vi "SVFA Power Spectrum Subset (1 Ch).vi"(0 "scaled signal [EU]":waveform(dbl)={"t0"=timestamp(0 s since 1904-01-01), "dt"=1e-05, "Y"=[]}, 2 "window":T7=1 items=["None"=0, "Hanning"=1, "Hamming"=2, "Blackman-Harris"=3, "Exact Blackman"=4, "Blackman"=5, "Flat Top"=6, "4 Term B-Harris "=7, "7 Term B-Harris"=8, "Low Sidelobe"=9, "Force"=64, "Exponential"=65, "Blackman Nuttall"=11, "Triangle"=30, "Bartlett-Hanning"=31, "Bohman"=32, "Parzen"=33, "Welch"=34, "Kaiser"=60, "Dolph-Chebyshev"=61, "Gaussian"=62], 3 "frequency range":T9={"start frequency"=1000.0, "stop frequency"=2000.0} {"stop frequency" min=0.0 format="%.2f"; "start frequency" min=0.0 format="%.2f"}, 4 "dB On (T)":bool=TRUE, 5 "error in (no error)":errorcluster, 7 "averaging parameters":T8={"averaging mode"=enum."No averaging", "weighting mode"=enum."Exponential", "number of averages"=10, "linear mode"=enum."One shot"}, 9 "restart averaging (F)":bool) -> (11 "averaging done":bool, 13 "averages completed":dbl, 14 "power spectrum [dB EU]":cluster{"f0":dbl, "df":dbl, "magnitude":dbl[]}={"f0"=nan, "df"=inf, "magnitude"=[]} {"magnitude" format="%.2p"; "df" format="%.2p"; "f0" format="%.2p"}, 15 "unit label":string, 18 "spectrum info":T1={"channel name"="", "description"="", "x-axis units"=1, "spectral info"={"spectrum type"=enum."Power [Magnitude^2]", "linear/dB"=enum."linear", "window"=0, "window size"=0, "FFT size"=0}, "engineering units"=0, "custom label"="", "dB reference [EU]"=0.0, "peak units"=enum."rms", "weighting filter"=0, "spectral density?"=FALSE, "unit label"="", "spectrum skewed?"=FALSE, "complimentary spectrum units"=enum."none"} {"x-axis units" items=["Time (s)"=0, "Frequency-CB (Hz)"=1, "Frequency-CPB (Hz)"=1248, "Frequency-Arbitrary (Hz)"=2357, "Quefrency (s)"=2, "Revolutions (rev)"=3, "Order"=4, "Speed (RPM)"=11, "Speed (rad/s)"=21, "Index"=65535]; "weighting filter" items=["Linear", "A-weighting", "B-weighting", "C-weighting", "ITU-R 468-4", "Dolby", "CCITT", "C-message", "Wb", "Wc", "Wd", "We", "Wf", "Wh", "Wj", "Wk", "Wm", "AES17 20 kHz lowpass", "AES17 40 kHz lowpass", "AES17 20 kHz highpass", "AES17 40 kHz highpass"]; "dB reference [EU]" format="%.2f"; "engineering units" items=["custom..."=0, "V"=1, "A"=21, "C"=30, "pC"=31, "s"=32, "-"=29, "Pa"=2, "N"=20, "g"=3, "m/s^2"=4, "m/s"=5, "m"=6, "mm/s"=12, "mm"=13, "micron/s"=14, "micron"=15, "in/s^2"=7, "in/s"=8, "in"=9, "mil/s"=10, "mil"=11, "rad/s^2"=16, "rad/s"=17, "rad"=18, "deg/s^2"=26, "deg/s"=27, "deg"=28, "RPM"=22, "cycle/s^2"=23, "Hz"=24, "cycle"=25, "strain"=19]; "spectral info"."window" items=["None "=0, "Hanning"=1, "Hamming"=2, "Blackman-Harris"=3, "Exact Blackman"=4, "Blackman"=5, "Flat Top"=6, "4 Term B-Harris "=7, "7 Term B-Harris"=8, "Low Sidelobe"=9, "Force - Exponential"=10, "Gaussian"=62]}, 19 "error out":errorcluster)   [LabVIEW 2017]
doc: "Computes a subset of the power spectrum of <B>scaled signal [EU]</B>. The subset is defined by <B>frequency range</B>. Each block of data corresponds to a single FFT block and has to be passed individually to this VI. Wire data to the <B>scaled signal [EU]</B> input to determine the polymorphic instance to use or manually select the instance."
uses:
  <vilib>/addons/_NISVFA/_Shared subVIs/Controls/svc_Window.ctl
  <vilib>/addons/_NISVFA/_Shared subVIs/Controls/svc_Spectrum Info.ctl
  <vilib>/addons/_NISVFA/_Shared subVIs/Controls/svc_X-Axis Units.ctl
  <vilib>/addons/_NISVFA/_Shared subVIs/Controls/svc_Spectrum Type.ctl
  <vilib>/addons/_NISVFA/_Shared subVIs/Controls/svc_Engineering Units Text Ring.ctl
  <vilib>/addons/_NISVFA/_Shared subVIs/Controls/svc_Weighting Filter Text Ring.ctl
  <vilib>/addons/_NISVFA/_Shared subVIs/Controls/svc_Complimentary Spectrum Units.ctl
  <vilib>/addons/_NISVFA/_Shared subVIs/Spectrum Averaging/svfa_Reset Averaging State Info.vi
  <vilib>/addons/_NISVFA/_Shared subVIs/Spectrum Averaging/svfa_Average Array with Avg Checks (complex) No State.vi
  <vilib>/addons/_NISVFA/_Shared subVIs/Common/svc_Complex to Mag2 Array.vi
  <vilib>/addons/_NISVFA/_Shared subVIs/Spectrum Averaging/svfa_Average Array with Avg Checks (real) No State.vi
  <vilib>/addons/_NISVFA/_Shared subVIs/Windowing/svfa_Scaled Time Domain Window (Array).vi
  <vilib>/addons/_NISVFA/_Shared subVIs/Common/svc_Get SV Channel Info.vi
  <vilib>/addons/_NISVFA/_Shared subVIs/Common/svc_Spectrum Units.vi
  <vilib>/addons/_NISVFA/_Shared subVIs/Spectrum Averaging/svfa_Average Array (complex) No State.vi
  <vilib>/addons/_NISVFA/_Shared subVIs/Spectrum Averaging/svfa_Average Array (real) No State.vi
  <vilib>/Analysis/4window.llb/Force Window.vi
  <vilib>/Analysis/4window.llb/Force Window (DBL).vi
  <vilib>/Analysis/4window.llb/Exponential Window.vi
  <vilib>/Analysis/4window.llb/Exponential Window (DBL).vi
  <vilib>/addons/_NISVFA/_Shared subVIs/Spectrum Averaging/svfa_No Average Array (complex).vi
  <vilib>/addons/_NISVFA/_Shared subVIs/Spectrum Averaging/svfa_Average Array (complex).vi
  <vilib>/addons/_NISVFA/_Shared subVIs/Spectrum Averaging/svfa_No Average Array (real).vi
  <vilib>/addons/_NISVFA/_Shared subVIs/Spectrum Averaging/svfa_Average Array (real).vi
  <vilib>/addons/_NISVFA/_Shared subVIs/Spectrum Averaging/svfa_Peak Hold Array.vi
  <vilib>/addons/_NISVFA/_Shared subVIs/Common/svc_Get Weighting Enum and Labels.vi
  <vilib>/addons/_NISVFA/_Shared subVIs/Common/svc_Unit Label Lexical Class.vi
  <vilib>/addons/_NISVFA/_Shared subVIs/Common/svc_Engineering Units to Unit Label.vi
  <vilib>/addons/_NISVFA/_Shared subVIs/Common/svc_Format Value (DBL).vi
  <vilib>/addons/_NISVFA/_Shared subVIs/Common/svc_Channel Info to Spectrum Info.vi
  <vilib>/addons/_NISVFA/_Shared subVIs/Common/svc_Unit Label to Engineering Units.vi
  <vilib>/Utility/error.llb/Error Cluster From Error Code.vi
  <vilib>/Analysis/0measdsp.llb/Scaled Time Domain Window.vi
  <vilib>/Analysis/0measdsp.llb/Scaled Time Domain Window (DBL).vi
  <vilib>/addons/_NISVFA/_Spectrum Processing/subVIs/svfa_Spectrum Info Window to windowTd Type Def.vi
  <vilib>/addons/_NISVFA/_Shared subVIs/Common/svc_Window Parameters.vi
  <vilib>/addons/_NISVFA/_Shared subVIs/Common/svc_Get Window Info.vi
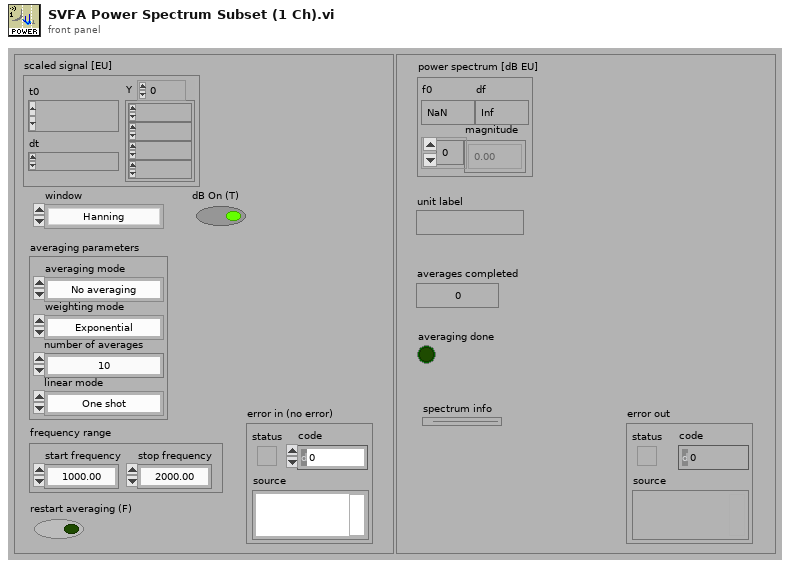
[diagram p1: front panel]
types:
  T1 = typedef "svc_Spectrum Info.ctl" = cluster{"channel name":string, "description":string, "x-axis units":T2, "spectral info":cluster{"spectrum type":T3, "linear/dB":enum16{"linear", "dB"}, "window":u16, "window size":i32, "FFT size":i32}, "engineering units":T4, "custom label":string, "dB reference [EU]":dbl, "peak units":enum16{"rms", "peak", "peak-peak"}, "weighting filter":T5, "spectral density?":bool, "unit label":string, "spectrum skewed?":bool, "complimentary spectrum units":T6}
  T2 = typedef "svc_X-Axis Units.ctl" = u16
  T3 = typedef "svc_Spectrum Type.ctl" = enum16{"FFT Spectrum [complex]", "Amplitude [Magnitude]", "Power [Magnitude^2]", "Cross Spectrum [complex]", "Frequency Response [Complex]"}
  T4 = typedef "svc_Engineering Units Text Ring.ctl" = u16
  T5 = typedef "svc_Weighting Filter Text Ring.ctl" = u16
  T6 = typedef "svc_Complimentary Spectrum Units.ctl" = enum16{"none", "radians", "degrees", "cycles", "imaginary"}
  T7 = typedef "svc_Window.ctl" = u32
  T8 = cluster{"averaging mode":enum16{"No averaging", "Vector averaging", "RMS averaging", "Peak hold"}, "weighting mode":enum16{"Linear", "Exponential"}, "number of averages":u32, "linear mode":enum16{"One shot", "Auto restart"}}
  T9 = cluster{"start frequency":dbl, "stop frequency":dbl}
  T10 = enum16{"Restart processing", "Continue processing", "Skip processing"}
  T11 = enum16{"No averaging", "Vector averaging", "RMS averaging", "Peak hold"}
  T12 = cluster{"complex FFT":cdb[], "real FFT":dbl[], "f0":dbl, "df":dbl, "averages completed":dbl, "averaging parameters":cluster{"averaging mode":enum16{"No averaging", "Vector averaging", "RMS averaging", "Peak hold"}, "weighting mode":enum16{"Linear", "Exponential"}, "number of averages":u32, "linear mode":enum16{"One shot", "Auto restart"}}}
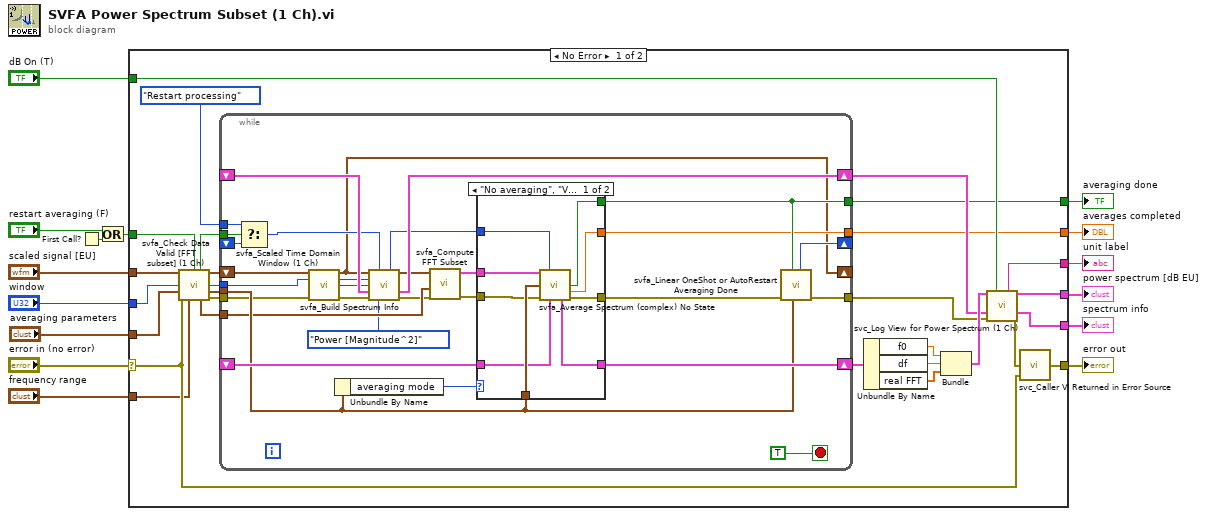
[diagram p0: block diagram]
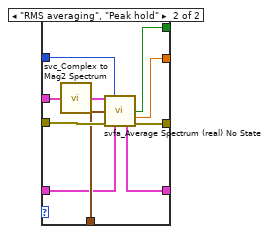
[diagram p2: hidden frame]
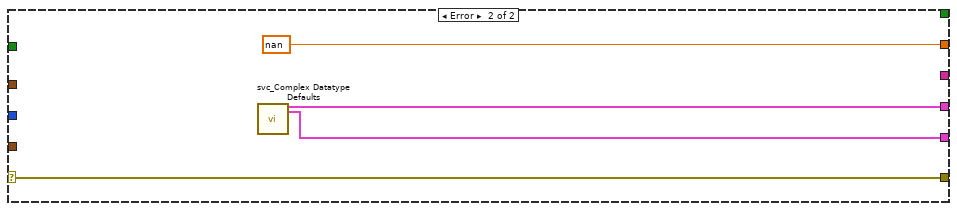
[diagram p3: hidden frame]
diagram:
  n1 = First Call?() -> (First Call?: T/F=w3:bool)
  n2 = Or(x="restart averaging (F)", y=w3) -> (x .or. y?=w2:bool)
  n3 = case shown="No Error" "error in (no error)" {
    selector: "error in (no error)" -> [w33 w96]
    tunnel: w2 -> [w41 _]
    tunnel: [w17 nan ("Averaged So-far")] -> w15
    tunnel: [w18 _] -> w14
    tunnel: [w38 w93] -> w9
    tunnel: [w35 w96] -> w13
    tunnel: "averaging parameters" -> [w40 _]
    tunnel: "frequency range" -> [w20 _]
    tunnel: "scaled signal [EU]" -> [w43 _]
    tunnel: "window" -> [w42 _]
    tunnel: [w37 _] -> w6
    tunnel: "dB On (T)" -> [w39 _]
    tunnel: [w34 w94] -> w4
    frame No Error {
      n4 = call <vilib>:"svfa_Check Data Valid [FFT subset] (1 Ch).vi"("signal"=w43, "restart averaging (F)"=w41, "window"=w42, "averaging parameters"=w40, "error in (no error)"=w33, "frequency range in"=w20) -> ("restart averaging"=w22:bool, "dup signal"=w28:waveform(dbl), "window"=w27:u16, "dup averaging parameters"=w24:T8, "frequency range out"=w19:T9, "error out"=w23:errorcluster)  [unwired: 4 in]
      n5 = while {
        shift-left: _ -> [w65]
        shift-right: [w66] -> w29
        tunnel: [w71] -> w17
        tunnel: [w72] -> w18
        tunnel: [w73] -> w16
        tunnel: w27 -> [w70]
        shift-right: [w68] -> w25
        shift-left: _ -> [w67]
        shift-right: [w64] -> _
        shift-left: _ -> [w63]
        tunnel: w24 -> [w61]
        tunnel: w23 -> [w60]
        tunnel: w22 -> [w59]
        tunnel: T10."Restart processing" ("t") -> [w58]
        tunnel: w19 -> [w57]
        shift-right: [w44] -> _
        shift-left: w28 -> [w45]
        stop <- TRUE stop-if-true
        n6 = Select(t=w58, s=w59, f=w63) -> (s? t:f=w62:T10)
        n7 = call <vilib>:"svfa_Scaled Time Domain Window (1 Ch).vi"("Signal in [X]"=w45, "window"=w70, "error in"=w60) -> ("Windowed Waveform"=w44:waveform(dbl), "dup window"=w49:T7, "window length"=w48:i32, "error out"=w50:errorcluster)  [unwired: 7 in, 2 out]
        n8 = Unbundle By Name(w61) -> ("averaging mode"=w56:T11)
        n9 = call <vilib>:"svfa_Build Spectrum Info.vi"("scaled signal [EU]"=w44, "processing control"=w62, "window"=w49, "window size"=w48, "spectrum info in"=w67, "error in (no error)"=w50, "spectrum type"=svc_Spectrum_Type."Power [Magnitude^2]" ("spectrum type 2")) -> ("dup processing control"=w47:T10, "dup scaled signal [EU]"=w46:waveform(dbl), "spectrum info out"=w68:T1, "error out"=w54:errorcluster)  [unwired: 5 in]
        n10 = call <vilib>:"svfa_Compute FFT Subset.vi"("error in (no error)"=w54, "frequency range"=w57, "windowed signal"=w46) -> ("error out"=w52:errorcluster, "FFT spectrum [Vrms]"=w51:cluster{"f0":dbl, "df":dbl, "spectrum":cdb[]})  [unwired: 7 in]
        n11 = case shown="\"No averaging\", \"Vector averaging\"" w56 {
          tunnel: w61 -> [w81 w86]
          tunnel: [w74 w83] -> w66
          tunnel: [w79 w90] -> w55
          tunnel: w51 -> [w82 w88]
          tunnel: w52 -> [w80 w92]
          tunnel: w47 -> [w76 w85]
          tunnel: [w77 w89] -> w71
          tunnel: w65 -> [w75 w84]
          tunnel: [w78 w91] -> w72
          frame "No averaging", "Vector averaging" {
            n12 = call <vilib>:"svfa_Average Spectrum (complex) No State.vi"("spectrum"=w82, "processing control"=w76, "averaging parameters"=w81, "error in (no error)"=w80, "averaging state info in"=w75) -> ("averaging done"=w78:bool, "averages completed"=w77:dbl, "averaging state info out"=w74:T12, "error out"=w79:errorcluster)  [unwired: 5 in, 2 out]
          }
          frame "RMS averaging", "Peak hold" {
            n13 = call <vilib>:"svc_Complex to Mag2 Spectrum.vi"("complex spectrum"=w88) -> ("power spectrum"=w87:cluster{"f0":dbl, "df":dbl, "spectrum":dbl[]})  [unwired: 4 in]
            n14 = call <vilib>:"svfa_Average Spectrum (real) No State.vi"("spectrum"=w87, "processing control"=w85, "averaging parameters"=w86, "error in (no error)"=w92, "averaging state info in"=w84) -> ("averaging done"=w91:bool, "averages completed"=w89:dbl, "averaging state info out"=w83:T12, "error out"=w90:errorcluster)  [unwired: 5 in, 2 out]
          }
        }
        n15 = call <vilib>:"svfa_Linear OneShot or AutoRestart Averaging Done.vi"("averaging parameters"=w61, "averaging done"=w72, "error in (no error)"=w55) -> ("error out"=w73:errorcluster, "processing control"=w64:T10)  [unwired: 7 in]
      }
      n16 = Unbundle By Name(w29) -> ("f0"=w32:dbl, "df"=w31:dbl, "real FFT"=w30:dbl[])
      n17 = Bundle("f0"=w32, "df"=w31, "real FFT"=w30) -> (w26:cluster{"f0":dbl, "df":dbl, "real FFT":dbl[]})  [unwired: 1 in]
      n18 = call <vilib>:"svc_Log View for Power Spectrum (1 Ch).vi"("power spectrum [dB EU]"=w26, "dB On (T)"=w39, "spectrum info"=w25, "error in (no error)"=w16) -> ("unit label"=w37:string, "power spectrum [dB EU]"=w38:cluster{"f0":dbl, "df":dbl, "magnitude":dbl[]}, "spectrum info out"=w34:T1, "error out"=w36:errorcluster)  [unwired: 8 in]
      n19 = call <vilib>:"svc_Caller VI Returned in Error Source.vi"("warning input to caller"=w33, "error in (no error)"=w36) -> ("error out"=w35:errorcluster)  [unwired: 3 in]
    }
    frame Error {
      n20 = call <vilib>:"svc_Complex Datatype Defaults.vi"() -> ("empty spectrum"=w93:cluster{"f0":dbl, "df":dbl, "magnitude":dbl[]}, "dead spectrum info"=w94:T1)  [unwired: 11 in, 7 out]
    }
  }
  "averages completed" <- w15
  "averaging done" <- w14
  "error out" <- w13
  "power spectrum [dB EU]" <- w9
  "unit label" <- w6
  "spectrum info" <- w4
